vi "MAIN_wQueue.vi"() -> ()   [LabVIEW 2016]
panel:
  out "Messages":i32(listbox)
  in  "STOP":bool
  in  "Start":bool
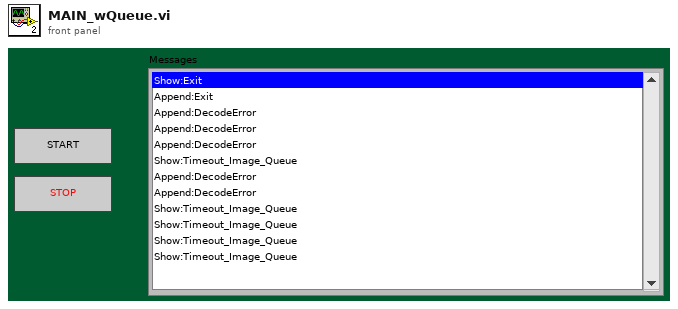
[diagram p1: front panel]
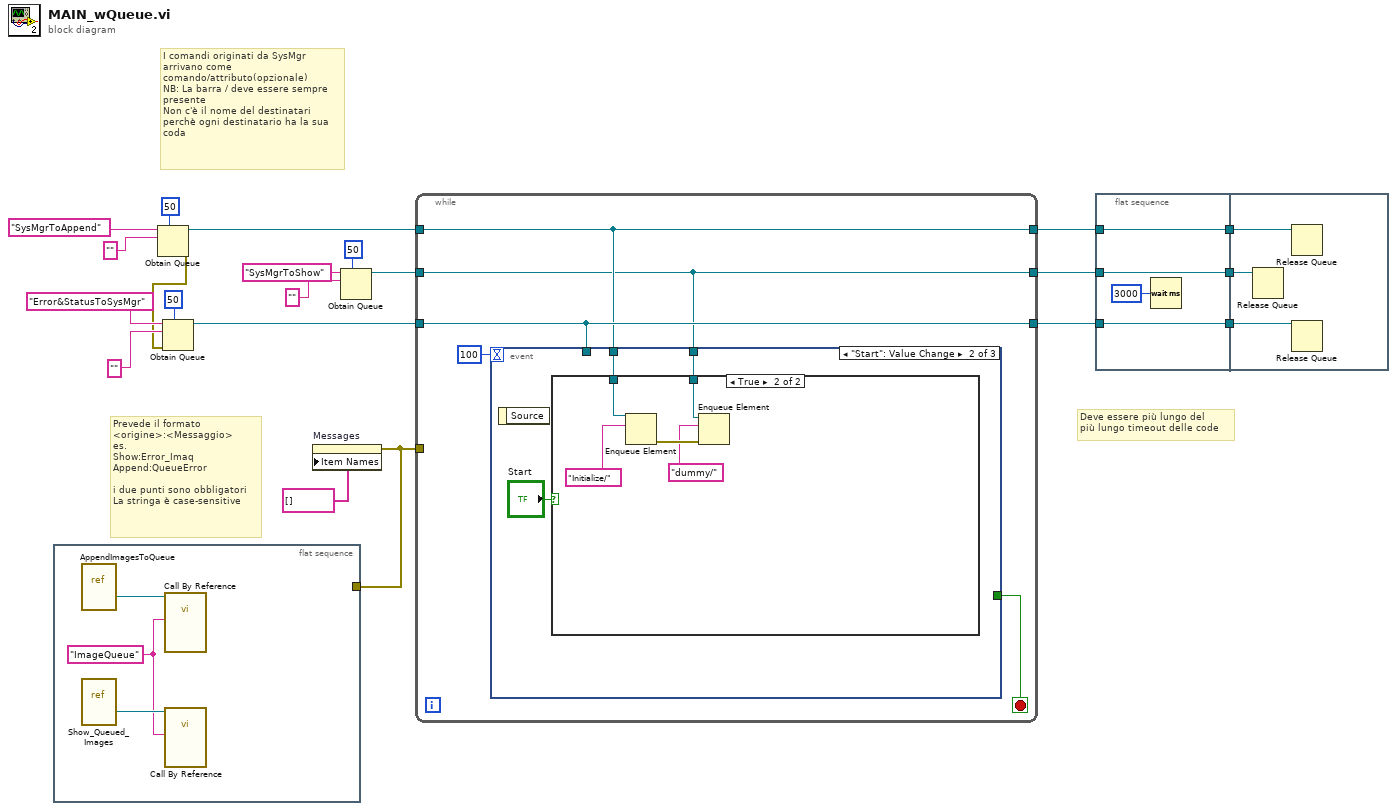
[diagram p0: block diagram]
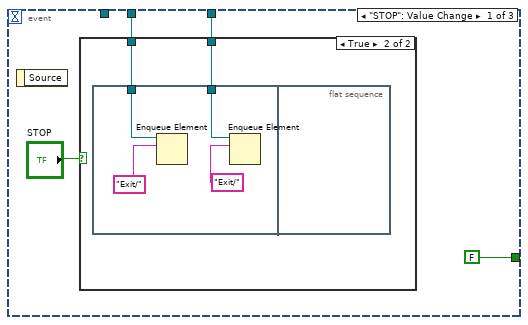
[diagram p2: hidden frame]
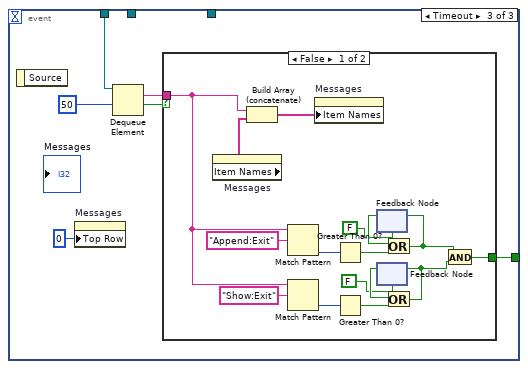
[diagram p5: hidden frame]
diagram:
  # "Deve essere più lungo del\npiù lungo timeout delle code"
  # "Prevede il formato\n<origine>:<Messaggio>\nes.\nShow:Error_Imaq\nAppend:QueueError\n\ni due punti sono obbligatori\nLa stringa è case-sensitive"
  # "I comandi originati da SysMgr \narrivano come\ncomando/attributo(opzionale)\nNB: La barra / deve essere sempre \npresente\nNon c'è il nome del destinatari\nperchè ogni destinatario ha la sua\ncoda"
  n1 = flat-sequence {
    tunnel: w1 -> [_]
    frame #0 {
      w22 = "ImageQueue" ("ImagesQueue")
      n2 = vi-ref "AppendImagesToQueue.vi"() -> (w24:refnum<vi>)
      n3 = vi-ref "Show_Queued_Images.vi"() -> (w23:refnum<vi>)
      n4 = call-by-ref "?"(reference=w24, "ImagesQueue"=w22) -> ()  [unwired: 11 in, 3 out]
      n5 = call-by-ref "?"(reference=w23, "ImagesQueue"=w22) -> ()  [unwired: 11 in, 3 out]
    }
  }
  n6 = Obtain Queue(max queue size (-1, unlimited)=50, name (unnamed)="SysMgrToAppend", element data type="") -> (queue out=w13:refnum<queue>, error out=w15:errorcluster)  [unwired: 2 in, 1 out]
  n7 = Obtain Queue(max queue size (-1, unlimited)=50, name (unnamed)="Error&StatusToSysMgr", element data type="", error in (no error)=w15) -> (queue out=w14:refnum<queue>)  [unwired: 1 in, 2 out]
  n8 = property on="Messages" class="LstBox (strict)"("Item Names"=string[] []) -> (error out=w1:errorcluster)  [unwired: 2 in, 1 out]
  n9 = Obtain Queue(max queue size (-1, unlimited)=50, name (unnamed)="SysMgrToShow", element data type="") -> (queue out=w7:refnum<queue>)  [unwired: 2 in, 2 out]
  n10 = while {
    tunnel: [w28] -> w11
    tunnel: w14 -> [w28]
    tunnel: [w27] -> w12
    tunnel: w13 -> [w27]
    tunnel: [w26] -> w6
    tunnel: w7 -> [w26]
    tunnel: w1 -> [_]
    stop <- w25 stop-if-true
    n11 = event shown="[1] \"Start\": Value Change" {
      selector: _ -> [_ _ _]
      dyn-events: _ -> [_ _ _]
      timeout: 100 -> [_ _ _]
      tunnel: w28 -> [_ _ w51]
      tunnel: w27 -> [w32 w41 _]
      tunnel: w26 -> [w31 w40 _]
      tunnel: [FALSE _ w49] -> w25
      event "STOP": Value Change {
        n12 = event-data() -> ()  [unwired: 1 in, 1 out]
        n13 = case shown="True" "STOP" {
          tunnel: w32 -> [_ w35]
          tunnel: w31 -> [_ w34]
          frame False {
          }
          frame True {
            n14 = flat-sequence {
              tunnel: w35 -> [w38]
              tunnel: w34 -> [w36]
              frame #0 {
                n15 = Enqueue Element(queue=w38, element="Exit/" ("notification")) -> ()  [unwired: 2 in, 3 out]
                n16 = Enqueue Element(queue=w36, element="Exit/" ("notification")) -> ()  [unwired: 2 in, 3 out]
              }
              frame #1 {
              }
            }
          }
        }
      }
      event "Start": Value Change {
        n17 = event-data() -> ()  [unwired: 1 in, 1 out]
        n18 = case shown="True" "Start" {
          tunnel: w41 -> [_ w44]
          tunnel: w40 -> [_ w43]
          frame False {
          }
          frame True {
            n19 = Enqueue Element(queue=w44, element="Initialize/" ("notification")) -> (error out=w46:errorcluster)  [unwired: 2 in, 2 out]
            n20 = Enqueue Element(queue=w43, element="dummy/" ("notification"), error in (no error)=w46) -> ()  [unwired: 1 in, 3 out]
          }
        }
      }
      event Timeout {
        n21 = event-data() -> ()  [unwired: 1 in, 1 out]
        n22 = property on="Messages" class="LstBox (strict)"("Top Row"=0) -> ()  [unwired: 2 in, 2 out]
        n23 = Dequeue Element(queue=w51, timeout in ms (-1)=50) -> (element=w50:string, timed out?=w52:bool)  [unwired: 1 in, 2 out]
        n24 = case shown="False" w52 {
          tunnel: w50 -> [w55 _]
          tunnel: [w54 _] -> w49
          frame False {
            n25 = property on="Messages" class="LstBox (strict)"() -> ("Item Names"=w69:string[])  [unwired: 2 in, 2 out]
            n26 = Build Array (concatenate)(w55, w69) -> (w68:string[])
            n27 = Match Pattern(string=w55, regular expression="Append:Exit") -> (offset past match=w65:i32)  [unwired: 1 in, 3 out]
            n28 = Match Pattern(string=w55, regular expression="Show:Exit") -> (offset past match=w61:i32)  [unwired: 1 in, 3 out]
            n29 = property on="Messages" class="LstBox (strict)"("Item Names"=w68) -> ()  [unwired: 2 in, 2 out]
            n30 = Greater Than 0?(x=w65) -> (x > 0?=w63:bool)
            n31 = Greater Than 0?(x=w61) -> (x > 0?=w62:bool)
            n32 = feedback #1(FALSE) -> (w64:bool)
            n33 = feedback #2(FALSE) -> (w60:bool)
            n34 = Or(x=w64, y=w63) -> (x .or. y?=w57:bool)
            n35 = feedback-in #1(w57) -> ()
            n36 = Or(x=w60, y=w62) -> (x .or. y?=w56:bool)
            n37 = feedback-in #2(w56) -> ()
            n38 = And(x=w57, y=w56) -> (x .and. y?=w54:bool)
          }
          frame True {
          }
        }
      }
    }
  }
  n39 = flat-sequence {
    tunnel: w6 -> [w71]
    tunnel: w11 -> [w72]
    tunnel: w12 -> [w73]
    tunnel: [w73] -> w5
    tunnel: [w72] -> w4
    tunnel: [w71] -> w3
    tunnel: w5 -> [w76]
    tunnel: w4 -> [w75]
    tunnel: w3 -> [w74]
    frame #0 {
      n40 = Wait (ms)(milliseconds to wait=u32 3000) -> ()  [unwired: 1 out]
    }
    frame #1 {
      n41 = Release Queue(queue=w74) -> ()  [unwired: 2 in, 3 out]
      n42 = Release Queue(queue=w76) -> ()  [unwired: 2 in, 3 out]
      n43 = Release Queue(queue=w75) -> ()  [unwired: 2 in, 3 out]
    }
  }
